vi "Prober_ReadXYZTheta.vi"(8 "error in (no error)":errorcluster, 11 "TeslaVeloxProbeStation in":refnum<class "TeslaVeloxProbeStation.lvclass">) -> (0 "error out":errorcluster, 1 "Z location [µm]":i32, 2 "Y location [µm]":i32, 3 "X location [µm]":i32, 4 "Theta location [mdeg]":i32, 5 "TeslaVeloxProbeStation out":refnum<class "TeslaVeloxProbeStation.lvclass">)   [LabVIEW 2018, in "TeslaVeloxProbeStation.lvclass"]
uses:
  TeslaVeloxProbeStation.lvclass
  TeslaVeloxProbeStation.lvclass/TeslaVeloxProbeStation.ctl
  Desktop/Kvasnicka/test_labview_library/Integration_toolkit_library/CascadeProbestation.lvlib
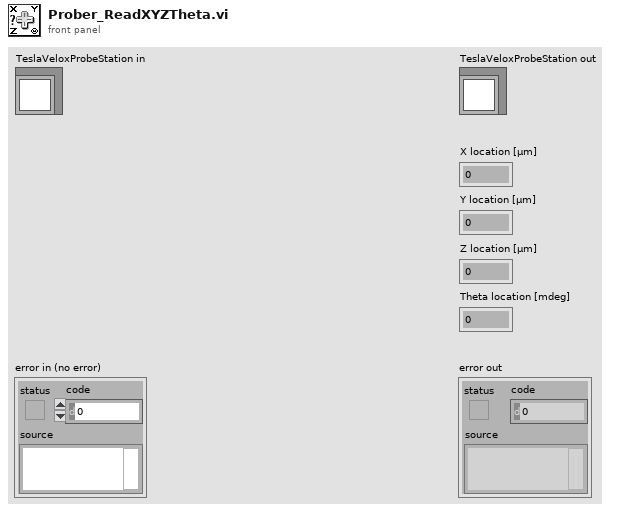
[diagram p1: front panel]
types:
  T1 = enum16{"Default", "Technology", "Offset", "Prober", "None"}
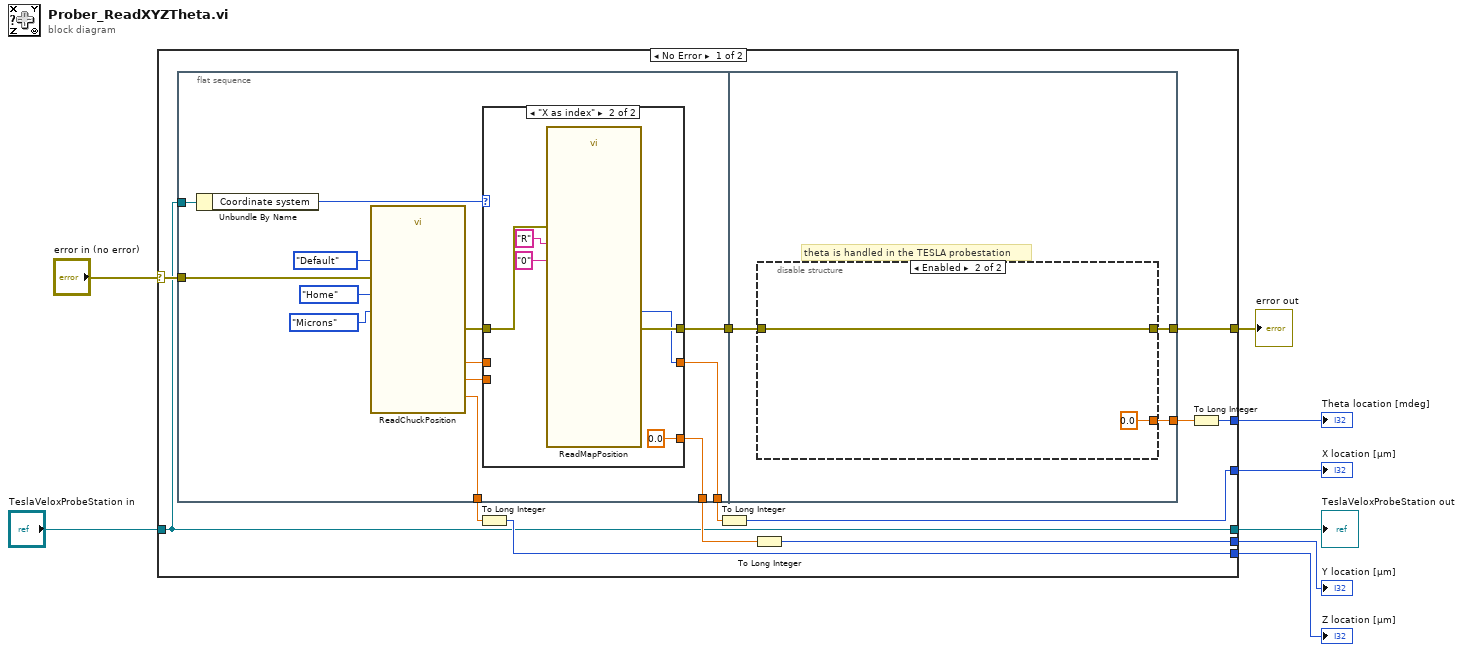
[diagram p0: block diagram]
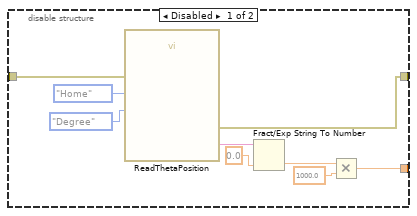
[diagram p3: hidden frame]
diagram:
  n1 = case shown="No Error" "error in (no error)" {
    selector: "error in (no error)" -> [w20 w58]
    tunnel: [w19 w58] -> w7
    tunnel: "TeslaVeloxProbeStation in" -> [w9 w57]
    tunnel: [w9 w57] -> w5
    tunnel: [w12 _] -> w4
    tunnel: [w14 _] -> w3
    tunnel: [w16 _] -> w2
    tunnel: [w10 _] -> w1
    frame No Error {
      n2 = flat-sequence {
        tunnel: w20 -> [w30]
        tunnel: [w21] -> w18
        tunnel: [w29] -> w17
        tunnel: [w23] -> w15
        tunnel: [w25] -> w13
        tunnel: w9 -> [w28]
        tunnel: [w44] -> w19
        tunnel: w18 -> [w45]
        tunnel: [w43] -> w11
        frame #0 {
          n3 = Unbundle By Name(w28) -> ("Coordinate system"=w27:enum16{"Cartesian", "X as index"})
          n4 = call "ReadChuckPosition.vi"("Unit"=enum16{"Microns", "Mils", "Index"}."Microns", "PosRef"=enum16{"Home", "Zero", "Center"}."Home", "CompLevel"=T1."Default", "Error In"=w30) -> ("X Value"=w26:dbl, "Y Value"=w24:dbl, "Z Value"=w29:dbl, "Error Out"=w22:errorcluster)  [unwired: 7 in, 1 out]
          n5 = case shown="\"X as index\"" w27 {
            tunnel: w26 -> [w36 _]
            tunnel: [w36 w38] -> w25
            tunnel: w24 -> [w35 _]
            tunnel: [w35 0.0 ("Y Value")] -> w23
            tunnel: w22 -> [w34 w42]
            tunnel: [w34 w41] -> w21
            frame "Cartesian", Default {
            }
            frame "X as index" {
              n6 = call "ReadMapPosition.vi"("Pos"="0", "FromPos"="R", "Error In"=w42) -> ("CurrentSubDie"=w38:i32, "Error Out"=w41:errorcluster)  [unwired: 15 in, 8 out]
            }
          }
        }
        frame #1 {
          # "theta is handled in the TESLA probestation"
          n7 = disable-structure shown="Enabled" {
            disable-tunnel: w45 -> [w54 w55]
            disable-tunnel: [w51 w55] -> w44
            disable-tunnel: [w49 0.0] -> w43
            frame Disabled {
              n8 = call "ReadThetaPosition.vi"("Error In"=w54, "PosRef"=enum16{"Home", "Zero", "Center"}."Home", "Unit"=enum16{"Degree", "Radian"}."Degree") -> ("Error Out"=w51:errorcluster, "Response"=w48:string)  [unwired: 7 in]
              n9 = Fract/Exp String To Number(string=w48, default (0 dbl)=0.0) -> (number=w46:dbl)  [unwired: 2 in, 1 out]
              n10 = Multiply(x=w46, y=1000.0) -> (x*y=w49:dbl)
            }
            frame Enabled {
            }
          }
        }
      }
      n11 = To Long Integer(number=w17) -> (32bit integer=w16:i32)
      n12 = To Long Integer(number=w13) -> (32bit integer=w12:i32)
      n13 = To Long Integer(number=w15) -> (32bit integer=w14:i32)
      n14 = To Long Integer(number=w11) -> (32bit integer=w10:i32)
    }
    frame Error {
    }
  }
  "error out" <- w7
  "X location [µm]" <- w4
  "Z location [µm]" <- w2
  "Theta location [mdeg]" <- w1
  "Y location [µm]" <- w3
  "TeslaVeloxProbeStation out" <- w5
